vi "DBL Resize Buffer.vi"(8 "error in (no error)":errorcluster, 11 "DBL Waveform Buffer in":refnum<class "DBL Waveform Buffer.lvclass">) -> (0 "error out":errorcluster, 3 "DBL Waveform Buffer out":refnum<class "DBL Waveform Buffer.lvclass">)   [LabVIEW 2015, in "DBL Waveform Buffer.lvclass"]
uses:
  DBL Waveform Buffer.lvclass
  Waveform Buffer/Waveform Buffer.lvclass/Waveform Buffer.ctl
  DBL Waveform Buffer.lvclass/DBL Waveform Buffer.ctl
  Waveform Buffer/Waveform Buffer.lvclass
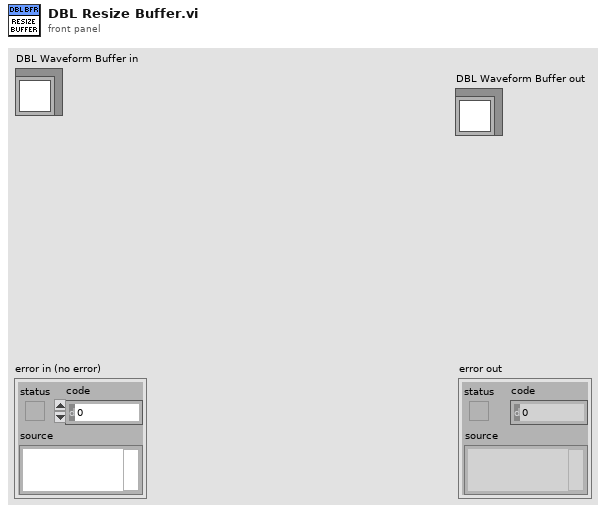
[diagram p1: front panel]
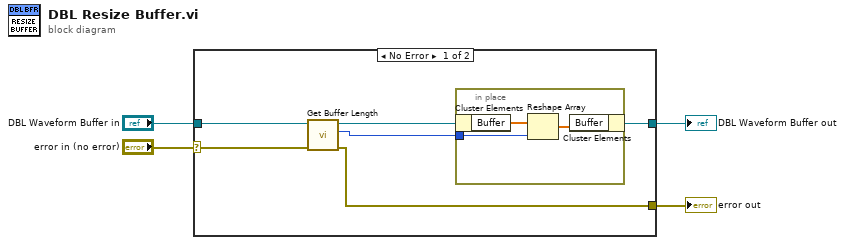
[diagram p0: block diagram]
diagram:
  n1 = case shown="No Error" "error in (no error)" {
    selector: "error in (no error)" -> [w7 w15]
    tunnel: [w6 w15] -> w2
    tunnel: [w8 w14] -> w1
    tunnel: "DBL Waveform Buffer in" -> [w10 w14]
    frame No Error {
      n2 = call "Get Buffer Length.vi"("error in (no error)"=w7, "Waveform Buffer in"=w10) -> ("error out"=w6:errorcluster, "Length"=w5:i32, "Waveform Buffer out"=w9:refnum<class "DBL Waveform Buffer.lvclass">)  [unwired: 7 in]
      n3 = in-place {
        in-place-border: w5 -> [w12]
        n4 = in-place-cluster #1(w9) -> ("Buffer"=w13:dbl[])
        n5 = Reshape Array(w13, w12) -> (w11:dbl[])
        n6 = in-place-cluster #1("Buffer"=w11) -> (w8:refnum<class "DBL Waveform Buffer.lvclass">)
      }
    }
    frame Error {
    }
  }
  "error out" <- w2
  "DBL Waveform Buffer out" <- w1
